vi "SAOMM-ROI_Fixer.vi"(0 "Binning":u16(ring)=5 items=["1 x 1"=1, "2 x 2"=2, "4 x 4"=4, "5 x 5"=5], 2 "Use Offset?":bool=TRUE, 5 "naxis":cluster{"Naxis1":u16, "Naxis2":u16}={"Naxis1"=1000, "Naxis2"=1000}, 7 "ROI":cluster{"ROIWidth":u16, "ROIYHeight":u16}={"ROIWidth"=80, "ROIYHeight"=80}, 9 "Offset":cluster{"ROIXOffset":u16, "ROIYOffset":u16}={"ROIXOffset"=950, "ROIYOffset"=950}, 11 "Reference Pixel":cluster{"PixelX":dbl, "PixelY":dbl}={"PixelX"=80.0, "PixelY"=80.0}) -> (4 "CoherenceError":bool, 8 "FixedROI":cluster{"ROIWidth":u16, "ROIYOffset":u16}, 10 "FixedOffset":cluster{"ROIXOffset":u16, "ROIYOffset":u16}, 15 "FixedPixel":cluster{"PixelX":dbl, "PixelY":dbl}={"PixelX"=80.0, "PixelY"=80.0})   [LabVIEW 2019]
panel:
  # "Offset"
  # "RefPix"
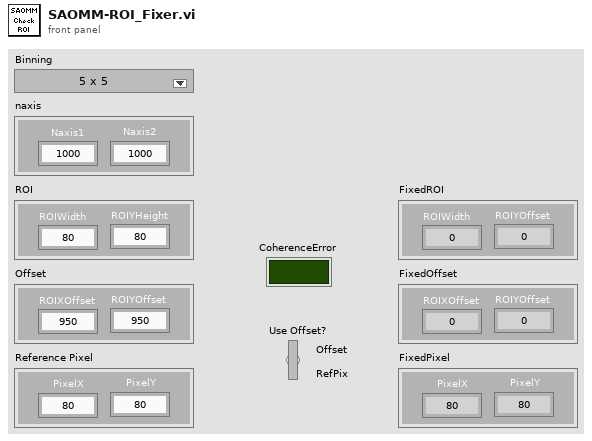
[diagram p1: front panel]
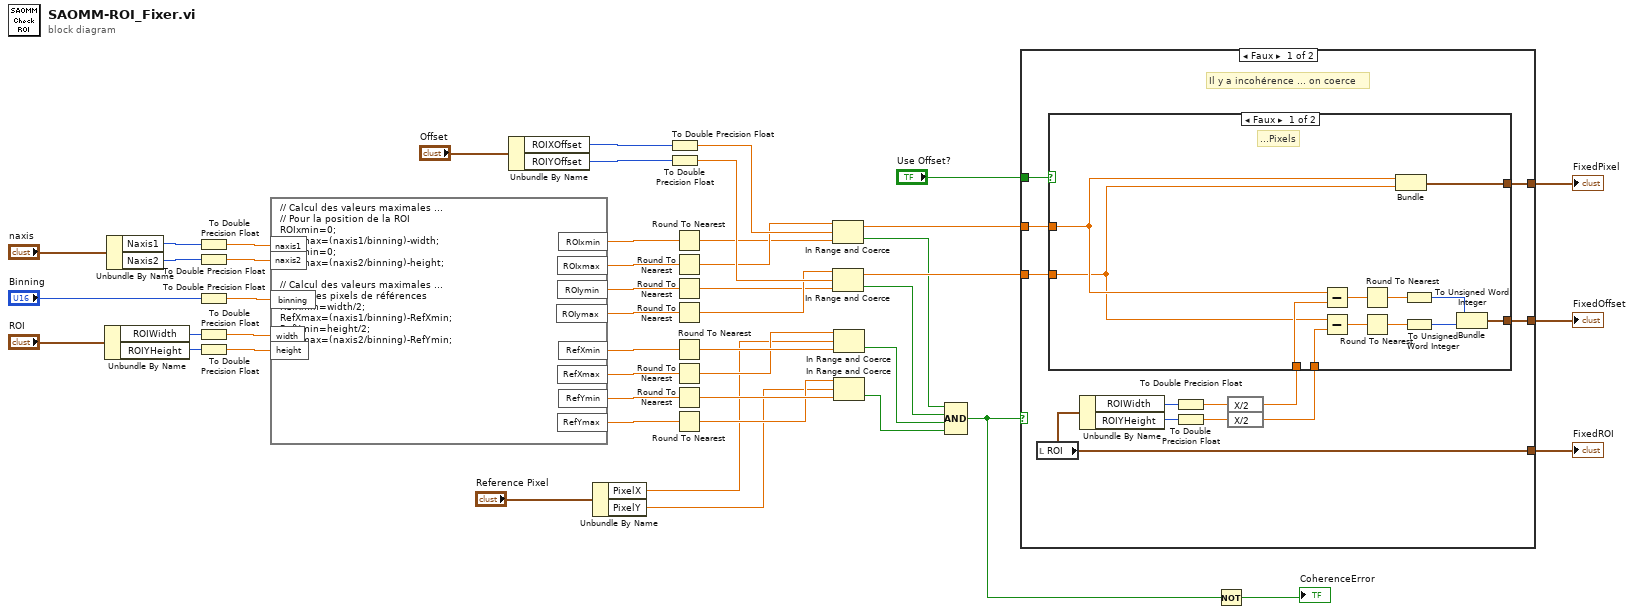
[diagram p0: block diagram]
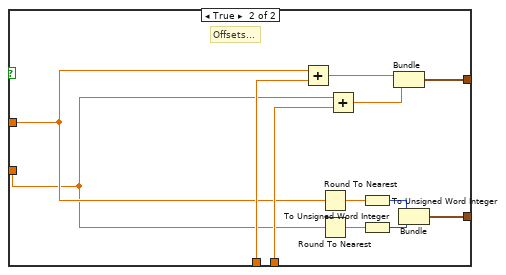
[diagram p2: hidden frame]
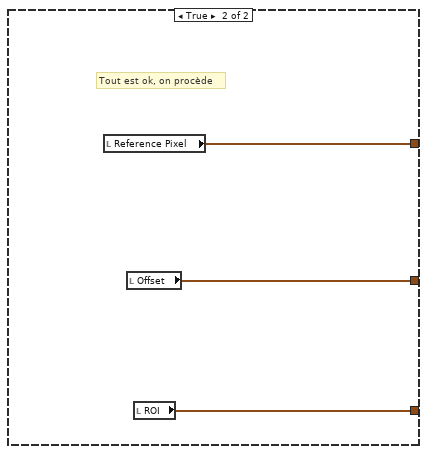
[diagram p3: hidden frame]
diagram:
  n1 = Unbundle By Name("ROI") -> ("ROIWidth"=w43:u16, "ROIYHeight"=w42:u16)
  n2 = Unbundle By Name("naxis") -> ("Naxis1"=w46:u16, "Naxis2"=w45:u16)
  n3 = To Double Precision Float(number=w46) -> (double precision float=w36:dbl)
  n4 = To Double Precision Float(number=w45) -> (double precision float=w37:dbl)
  n5 = To Double Precision Float(number="Binning") -> (double precision float=w38:dbl)
  n6 = To Double Precision Float(number=w43) -> (double precision float=w39:dbl)
  n7 = To Double Precision Float(number=w42) -> (double precision float=w40:dbl)
  n8 = formula code="// Calcul des valeurs maximales ...\n// Pour la position de la ROI\nROIxmin=0;\nROIxmax=(naxis1/binning)-width;\nROIymin=0;\nROIymax=(naxis2/binning)-height;\n\n// Calcul des valeurs maximales ...\n// Pour les pixels de références\nRefXmin=width/2;\nRefXmax=(naxis1/binning)-RefXmin;\nRefYmin=height/2;\nRefYmax=(naxis2/binning)-RefYmin;"("naxis1"=w36, "naxis2"=w37, "binning"=w38, "width"=w39, "height"=w40) -> ("ROIxmin"=w32:dbl, "ROIxmax"=w35:dbl, "ROIymin"=w34:dbl, "ROIymax"=w33:dbl, "RefXmin"=w14:dbl, "RefYmax"=w11:dbl, "RefXmax"=w13:dbl, "RefYmin"=w12:dbl)
  n9 = Unbundle By Name("Offset") -> ("ROIXOffset"=w16:u16, "ROIYOffset"=w15:u16)
  n10 = Unbundle By Name("Reference Pixel") -> ("PixelX"=w6:dbl, "PixelY"=w5:dbl)
  n11 = To Double Precision Float(number=w16) -> (double precision float=w28:dbl)
  n12 = To Double Precision Float(number=w15) -> (double precision float=w27:dbl)
  n13 = Round To Nearest(number=w32) -> (nearest integer value=w17:dbl)
  n14 = Round To Nearest(number=w35) -> (nearest integer value=w18:dbl)
  n15 = Round To Nearest(number=w34) -> (nearest integer value=w19:dbl)
  n16 = Round To Nearest(number=w33) -> (nearest integer value=w20:dbl)
  n17 = Round To Nearest(number=w14) -> (nearest integer value=w10:dbl)
  n18 = Round To Nearest(number=w13) -> (nearest integer value=w7:dbl)
  n19 = Round To Nearest(number=w12) -> (nearest integer value=w9:dbl)
  n20 = Round To Nearest(number=w11) -> (nearest integer value=w8:dbl)
  n21 = In Range and Coerce(upper limit=w18, x=w28, lower limit=w17) -> (coerced(x)=w30:dbl, In Range?=w1:bool)
  n22 = In Range and Coerce(upper limit=w20, x=w27, lower limit=w19) -> (coerced(x)=w29:dbl, In Range?=w2:bool)
  n23 = In Range and Coerce(upper limit=w7, x=w6, lower limit=w10) -> (In Range?=w3:bool)  [unwired: 1 out]
  n24 = In Range and Coerce(upper limit=w8, x=w5, lower limit=w9) -> (In Range?=w4:bool)  [unwired: 1 out]
  n25 = Compound Arithmetic op=AND(w1, w2, w3, w4) -> (w23:bool)
  n26 = case shown="Faux" w23 {
    tunnel: w30 -> [w60 _]
    tunnel: w29 -> [w59 _]
    tunnel: [w55 w87] -> w26
    tunnel: [w58 w86] -> w25
    tunnel: [w56 w85] -> w22
    tunnel: "Use Offset?" -> [w57 _]
    frame False {
      # "Il y a incohérence ... on coerce"
      n27 = local read "ROI"() -> (w55:cluster{"ROIWidth":u16, "ROIYHeight":u16})
      n28 = Unbundle By Name(w55) -> ("ROIWidth"=w53:u16, "ROIYHeight"=w54:u16)
      n29 = To Double Precision Float(number=w53) -> (double precision float=w50:dbl)
      n30 = To Double Precision Float(number=w54) -> (double precision float=w49:dbl)
      n31 = expression code="X/2"(w50) -> (w52:dbl)
      n32 = expression code="X/2"(w49) -> (w51:dbl)
      n33 = case shown="Faux" w57 {
        tunnel: w60 -> [w66 w74]
        tunnel: w59 -> [w65 w73]
        tunnel: [w71 w84] -> w58
        tunnel: [w72 w83] -> w56
        tunnel: w52 -> [w68 w81]
        tunnel: w51 -> [w69 w79]
        frame False {
          # "...Pixels"
          n34 = Subtract(x=w66, y=w68) -> (x-y=w67:dbl)
          n35 = Subtract(x=w65, y=w69) -> (x-y=w70:dbl)
          n36 = Round To Nearest(number=w67) -> (nearest integer value=w64:dbl)
          n37 = Round To Nearest(number=w70) -> (nearest integer value=w62:dbl)
          n38 = Bundle(w66, w65) -> (w72:cluster{dbl, dbl})  [unwired: 1 in]
          n39 = To Unsigned Word Integer(number=w64) -> (unsigned 16bit integer=w63:u16)
          n40 = To Unsigned Word Integer(number=w62) -> (unsigned 16bit integer=w61:u16)
          n41 = Bundle(w63, w61) -> (w71:cluster{u16, u16})  [unwired: 1 in]
        }
        frame True {
          # "Offsets..."
          n42 = Add(x=w74, y=w81) -> (x+y=w82:dbl)
          n43 = Round To Nearest(number=w74) -> (nearest integer value=w78:dbl)
          n44 = Round To Nearest(number=w73) -> (nearest integer value=w77:dbl)
          n45 = Add(x=w73, y=w79) -> (x+y=w80:dbl)
          n46 = To Unsigned Word Integer(number=w78) -> (unsigned 16bit integer=w75:u16)
          n47 = To Unsigned Word Integer(number=w77) -> (unsigned 16bit integer=w76:u16)
          n48 = Bundle(w82, w80) -> (w83:cluster{dbl, dbl})  [unwired: 1 in]
          n49 = Bundle(w75, w76) -> (w84:cluster{u16, u16})  [unwired: 1 in]
        }
      }
    }
    frame True {
      # "Tout est ok, on procède"
      n50 = local read "Reference Pixel"() -> (w85:cluster{"PixelX":dbl, "PixelY":dbl})
      n51 = local read "Offset"() -> (w86:cluster{"ROIXOffset":u16, "ROIYOffset":u16})
      n52 = local read "ROI"() -> (w87:cluster{"ROIWidth":u16, "ROIYHeight":u16})
    }
  }
  "FixedOffset" <- w25
  "FixedROI" <- w26
  "FixedPixel" <- w22
  n53 = Not(x=w23) -> (.not. x?=→"CoherenceError":bool)
